vi "Step of Adv params.vi"(7 "Step of ADV params":T1, 8 "error in (no error)":errorcluster, 10 "Step NO":u8=1 min=1 max=50 step=1, 11 "Profile NO":u8=1 min=1 max=50 step=1) -> (0 "error out":errorcluster, 2 "wchitch params":string, 3 "params array out":string[](array[string]))   [LabVIEW 2019, in "STAV lib.lvlib"]
uses:
  STAV lib.lvlib
  Step of Adv params.ctl
  Param Direction.ctl
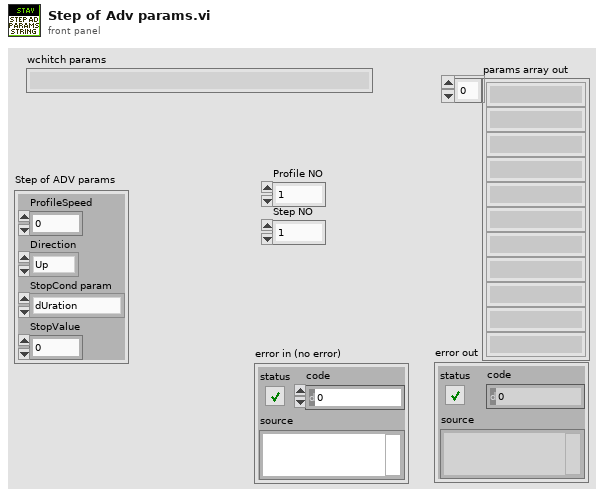
[diagram p1: front panel]
types:
  T1 = typedef "STAV lib.lvlib/Step of Adv params.ctl" = cluster{"ProfileSpeed":dbl, "Direction":T2, "StopCond param":enum16{"dUration", "dIstance", "Position", "force Greater", "force Smaller", "Break", "keep Force"}, "StopValue":dbl}
  T2 = typedef "STAV lib.lvlib/Param Direction.ctl" = enum16{"Up", "Down", "Left", "Right"}
  T3 = enum16{"dUration", "dIstance", "Position", "force Greater", "force Smaller", "Break", "keep Force"}
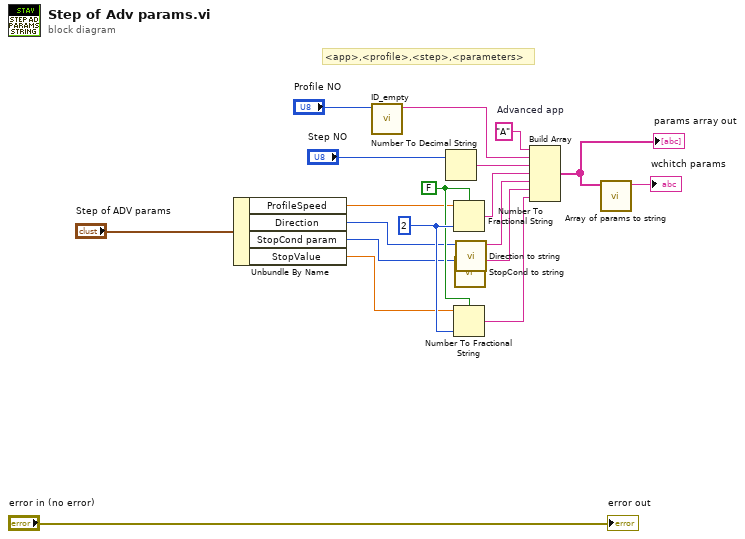
[diagram p0: block diagram]
diagram:
  w16 = i16 2 ("precision (6)")
  w15 = FALSE ("use system decimal point (T)")
  w19 = "A"  # Advanced app
  # "<app>,<profile>,<step>,<parameters>"
  n1 = Unbundle By Name("Step of ADV params") -> ("ProfileSpeed"=w7:dbl, "Direction"=w6:T2, "StopCond param"=w4:T3, "StopValue"=w1:dbl)
  n2 = call "ID_empty.vi"("Profile NO"="Profile NO") -> ("Profile NO out"=w14:string)  [unwired: 9 in, 1 out]
  n3 = Number To Decimal String(number="Step NO") -> (decimal integer string=w9:string)  [unwired: 1 in]
  n4 = Number To Fractional String(use system decimal point (T)=w15, number=w7, precision (6)=w16) -> (F-format string=w8:string)  [unwired: 1 in]
  n5 = Number To Fractional String(use system decimal point (T)=w15, number=w1, precision (6)=w16) -> (F-format string=w2:string)  [unwired: 1 in]
  n6 = call "StopCond to string.vi"("StopCond param"=w4) -> ("String"=w3:string)  [unwired: 10 in]
  n7 = call "Direction to string.vi"("Direction"=w6) -> ("Peak app"=w5:string)  [unwired: 10 in]
  n8 = Build Array(w19, w14, w9, w8, w5, w3, w2) -> (w13:string[])
  "params array out" <- w13
  n9 = call "Array of params to string.vi"("Array"=w13) -> ("String"=→"wchitch params":string)  [unwired: 10 in]
  "error out" <- "error in (no error)"
